vi "jacobi(SubVI).vi"(4 "Tolerancja":dbl, 8 "Initiial Guess":dbl[](array[numeric]), 10 "b":dbl[](array[numeric]), 11 "A":dbl[][](array[numeric])) -> (2 "Wykonana iczba Iteracji":i32, 3 "Metoda Jacobiego":dbl[](array[numeric]))   [LabVIEW 2020]
uses:
  <vilib>/Analysis/Matrix/Numeric/Conversions/Array To Matrix - RA2.vi
  <vilib>/Analysis/Matrix/Numeric/Conversions/Array To Matrix - RA.vi
  <vilib>/addons/Multicore Analysis and Sparse Matrix/Linear Algebra/_linalg/Inverse Matrix (DBL).vi
  <vilib>/Analysis/BLAS.llb/dgemv - General Matrix-Vector Product (DBL).vi
  <vilib>/Analysis/Matrix/Numeric/Multiply/Multiply - RM,R.vi
  <vilib>/Analysis/Matrix/Numeric/Multiply/Multiply - RM,RM.vi
  <vilib>/addons/Multicore Analysis and Sparse Matrix/BLAS/_blas/dgemv - General Matrix-Vector Product (DBL).vi
  <vilib>/Analysis/Matrix/NI_Matrix.lvlib
  <vilib>/addons/Multicore Analysis and Sparse Matrix/BLAS/NI_MASM_BLAS.lvlib
  <vilib>/Analysis/NI_AALBLAS.lvlib
  <vilib>/addons/Multicore Analysis and Sparse Matrix/Linear Algebra/NI_MASM_BasicLinAlg.lvlib
panel:
  out "Wczesny stop":bool
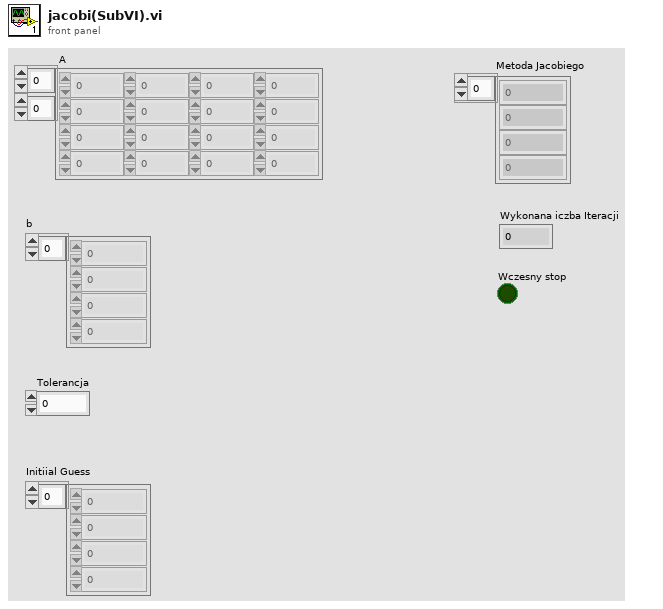
[diagram p1: front panel]
types:
  T1 = typedef "NI_Matrix.lvlib/RealMatrix.ctl" = dbl[][]
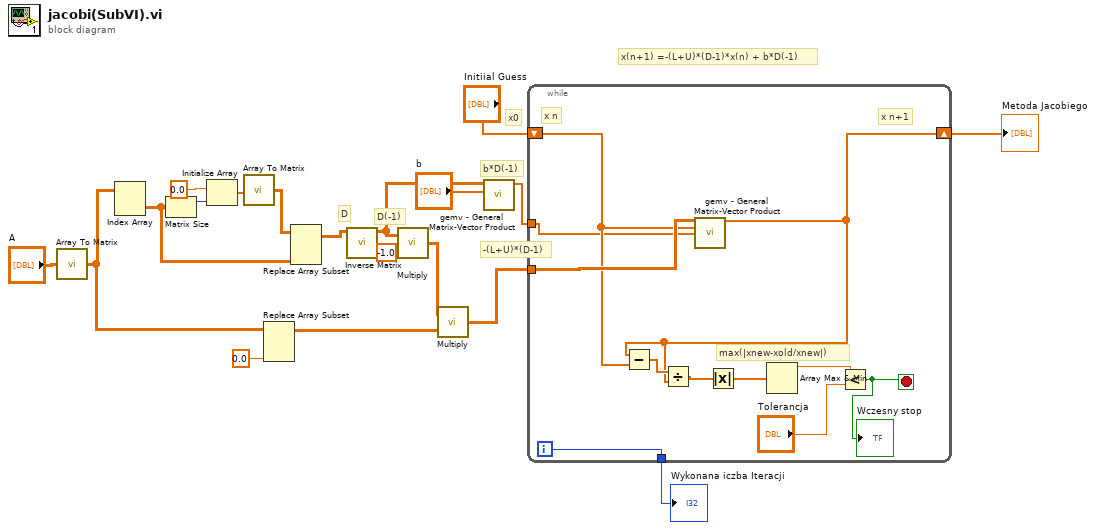
[diagram p0: block diagram]
diagram:
  # "x(n+1) =-(L+U)*(D-1)*x(n) + b*D(-1)"
  # "D(-1)"
  # "D"
  # "-(L+U)*(D-1)"
  # "x0"
  # "b*D(-1)"
  n1 = call-poly <vilib>:"Array To Matrix.vi"("Real 2D Array"="A") -> ("Real Matrix"=w14:T1)
  n2 = Index Array(array=w14) -> (element=w6:T1)  [unwired: 2 in]
  n3 = Matrix Size(0:w6) -> (1:w11:i32)  [unwired: 1 out]
  n4 = Initialize Array(0.0 ("element"), w11) -> (w9:dbl[])
  n5 = call-poly <vilib>:"Array To Matrix.vi"("Real 1D Array"=w9) -> ("Real Matrix (Column Vector)"=w8:T1)
  n6 = Replace Array Subset(array=w14, new element=0.0 ("new diagonal/fill element")) -> (w1:T1)  [unwired: 2 in]
  n7 = Replace Array Subset(array=w8, new element=w6) -> (w7:T1)  [unwired: 2 in]
  n8 = call-poly <vilib>:"Inverse Matrix.vi"("Input Matrix"=w7) -> ("Inverse Matrix"=w2:T1)  [unwired: 9 in, 1 out]
  n9 = call-poly <vilib>:"Multiply.vi"("Real Scalar c"=-1.0 ("y"), "Real Matrix A"=w2) -> ("A * c"=w12:T1)
  n10 = call-poly <vilib>:"Multiply.vi"("Real Matrix B"=w1, "Real Matrix A"=w12) -> ("A * B"=w3:T1)
  n11 = call-poly <vilib>:"gemv - General Matrix-Vector Product.vi"("x"="b", "A"=w2) -> ("dgemv"=w17:dbl[])  [unwired: 8 in, 1 out]
  n12 = while {
    tunnel: w17 -> [w20]
    shift-right: [w23] -> w19
    shift-left: "Initiial Guess" -> [w21]
    tunnel: w3 -> [w22]
    tunnel: [w25] -> w15
    i -> [w25]
    stop <- w24 stop-if-true
    # "max(|xnew-xold/xnew|)"
    # "x n"
    # "x n+1"
    n13 = call-poly <vilib>:"gemv - General Matrix-Vector Product.vi"("A"=w22, "x"=w21, "y"=w20) -> ("dgemv"=w23:dbl[])  [unwired: 11 in, 1 out]
    n14 = Subtract(x=w23, y=w21) -> (x-y=w30:dbl[])
    n15 = Divide(x=w30, y=w23) -> (x/y=w29:dbl[])
    n16 = Absolute Value(x=w29) -> (abs(x)=w28:dbl[])
    n17 = Array Max & Min(array=w28) -> (max value=w27:dbl)  [unwired: 3 out]
    n18 = Less?(x=w27, y="Tolerancja") -> (x < y?=w24:bool)
    "Wczesny stop" <- w24
  }
  "Metoda Jacobiego" <- w19
  "Wykonana iczba Iteracji" <- w15
